vi "GEN_Colors_positions.vi"(2 "Highest color position":u32, 3 "Initial colors ramp array in":T1) -> (0 "Colors positions":dbl[](array[numeric]), 1 "Initial colors ramp array out":T1)   [LabVIEW 2018, in "Tracker.lvlib"]
uses:
  Tracker.lvlib
  Controls/CTL_Color_ramp.ctl
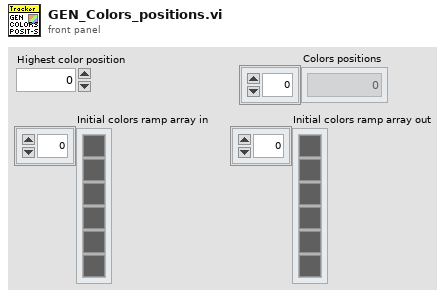
[diagram p1: front panel]
types:
  T1 = typedef "Tracker.lvlib/CTL_Color_ramp.ctl" = u32[]
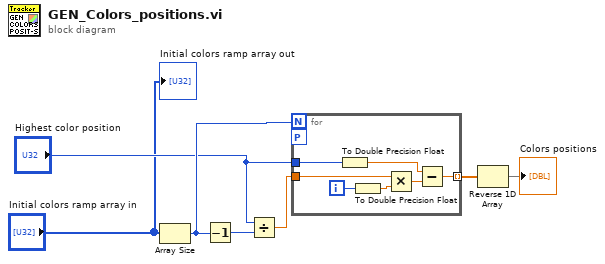
[diagram p0: block diagram]
diagram:
  n1 = Array Size(array="Initial colors ramp array in") -> (size(s)=w7:i32)
  n2 = Decrement(x=w7) -> (x-1=w4:i32)
  n3 = Divide(x="Highest color position", y=w4) -> (x/y=w3:dbl)
  n4 = for {
    N: w7 -> [_]
    tunnel: [w10] -> w5 mode=indexing
    tunnel: "Highest color position" -> [w14]
    tunnel: w3 -> [w12]
    workers-P: _ -> [_]
    i -> [w11]
    n5 = To Double Precision Float(number=w14) -> (double precision float=w9:dbl)
    n6 = To Double Precision Float(number=w11) -> (double precision float=w8:dbl)
    n7 = Multiply(x=w12, y=w8) -> (x*y=w13:dbl)
    n8 = Subtract(x=w9, y=w13) -> (x-y=w10:dbl)
  }
  n9 = Reverse 1D Array(array=w5) -> (reversed array=→"Colors positions":dbl[])
  "Initial colors ramp array out" <- "Initial colors ramp array in"
